vi "SSM2603 Write Register.vi"(8 "Error In (No Error)":errorcluster, 9 "Reg Data":u16 format="b%09b", 10 "Reg Address":u8, 11 "FPGA VI Reference In":T1) -> (0 "error out":errorcluster, 3 "FPGA VI Reference Out":T1)   [LabVIEW 2015]
uses:
  DSDB FPGA Ref.ctl
panel:
  # "Overview: This VI use I2C to write SSM2603 registers. SSM2603 use 9-bit registers to configure chip."
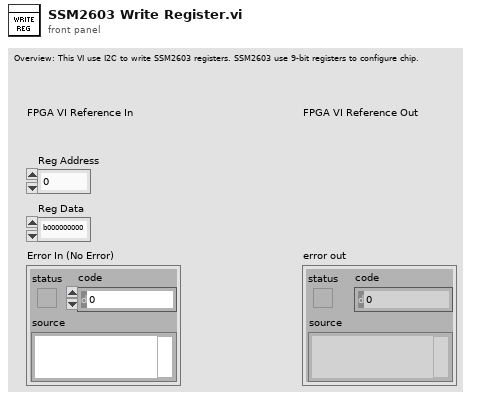
[diagram p1: front panel]
types:
  T1 = typedef "DSDB FPGA Ref.ctl" = refnum<k20>
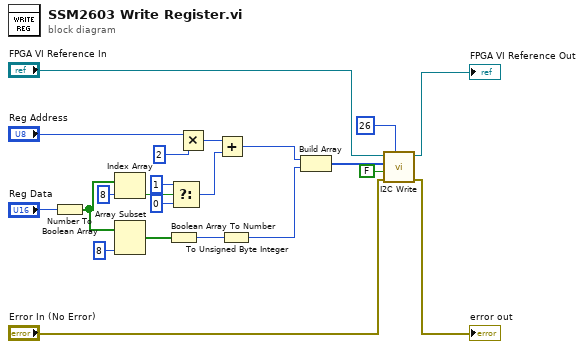
[diagram p0: block diagram]
diagram:
  n1 = Number To Boolean Array(number="Reg Data") -> (Boolean array=w8:bool[])
  n2 = Index Array(array=w8, index=8) -> (element=w15:bool)
  n3 = Array Subset(array=w8, length=8) -> (w6:bool[])  [unwired: 1 in]
  n4 = Boolean Array To Number(Boolean array=w6) -> (number=w5:u32)
  n5 = Select(t=u8 1, s=w15, f=u8 0) -> (s? t:f=w12:u8)
  n6 = Multiply(x="Reg Address", y=u8 2) -> (x*y=w13:u8)
  n7 = Add(x=w13, y=w12) -> (x+y=w4:u8)
  n8 = To Unsigned Byte Integer(number=w5) -> (unsigned 8bit integer=w3:u8)
  n9 = Build Array(w4, w3) -> (w2:u8[])
  n10 = call "I2C Write.vi"("Slave Address (7-bit)"=u8 26, "Error In (No Error)"="Error In (No Error)", "Keep Bus Busy"=FALSE, "Data to Write"=w2, "FPGA VI Reference In"="FPGA VI Reference In") -> ("error out"=→"error out":errorcluster, "FPGA VI Reference Out"=→"FPGA VI Reference Out":T1)  [unwired: 5 in]
